vi "Pointer.Write (1D U8).vi"(8 "error in (no error)":errorcluster, 10 "values":u8[](array[numeric]), 11 "pointer in":u64) -> (0 "error out":errorcluster, 2 "values out":u8[](array[numeric]), 3 "pointer out":u64)   [LabVIEW 2016, in "VeriStand Data.lvlib"]
doc: "Writes the contents of the provided <B>values</B> array to the memory location specified by <B>pointer</B>."
uses:
  VeriStand Data.lvlib
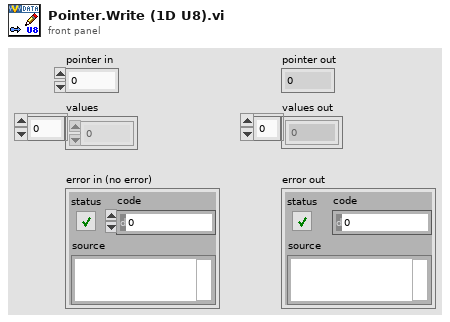
[diagram p1: front panel]
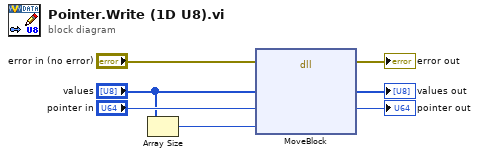
[diagram p0: block diagram]
diagram:
  n1 = Array Size(array="values") -> (size(s)=w1:i32)
  n2 = dll-call lib="LabVIEW" fn="MoveBlock"(error in="error in (no error)", "ps"="values", "pd"="pointer in", "size"=w1) -> (error out=→"error out":errorcluster, "ps"=→"values out":u8[], "pd"=→"pointer out":u64)  [unwired: 4 in, 1 out]
